vi "Main.vi"() -> ()   [LabVIEW 2017]
uses:
  47dd9ab8-544f-4192-a7de-fb61588ea7e2.vi
panel:
  out "Thermometer m6":dbl(slide) scale=10.0..50.0
  out "Thermometer m5":dbl(slide) scale=10.0..50.0
  out "Thermometer m3":dbl(slide) scale=10.0..50.0
  out "Thermometer m2":dbl(slide) scale=10.0..50.0
  out "Load m6":dbl(knob) scale=0.0..50.0
  out "Load m5":dbl(knob) scale=0.0..50.0
  out "Load m3":dbl(knob) scale=0.0..50.0
  out "Load m2":dbl(knob) scale=0.0..50.0
  out "error out":errorcluster
  in  "error in (no error)":errorcluster
  in  "Color m6":T1(ring)
  in  "Color m5":T1(ring)
  in  "Color m3":T1(ring)
  in  "Color m2":T1(ring)
  in  "Speed m6":dbl(slide)=1.0 scale=0.2..2.0
  in  "Speed m5":dbl(slide)=1.0 scale=0.2..2.0
  in  "Speed m3":dbl(slide)=1.0 scale=0.2..2.0
  in  "Speed m2":dbl(slide)=1.0 scale=0.2..2.0
  in  "m6":dbl(knob) scale=-23.0..90.0
  in  "m5":dbl(knob) scale=-90.0..90.0
  in  "m3":dbl(knob) scale=-90.0..90.0
  in  "m2":dbl(knob) scale=-90.0..90.0
  in  "stop":bool
  out "Picture":picture
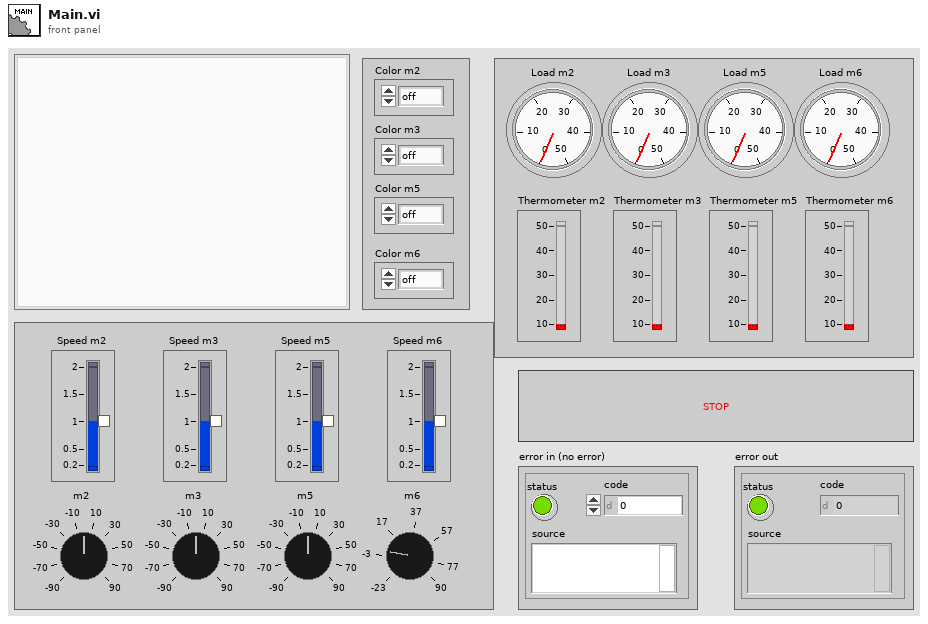
[diagram p1: front panel]
types:
  T1 = enum16{"off", "red", "green", "yellow", "blue", "pink", "cyan", "white"}
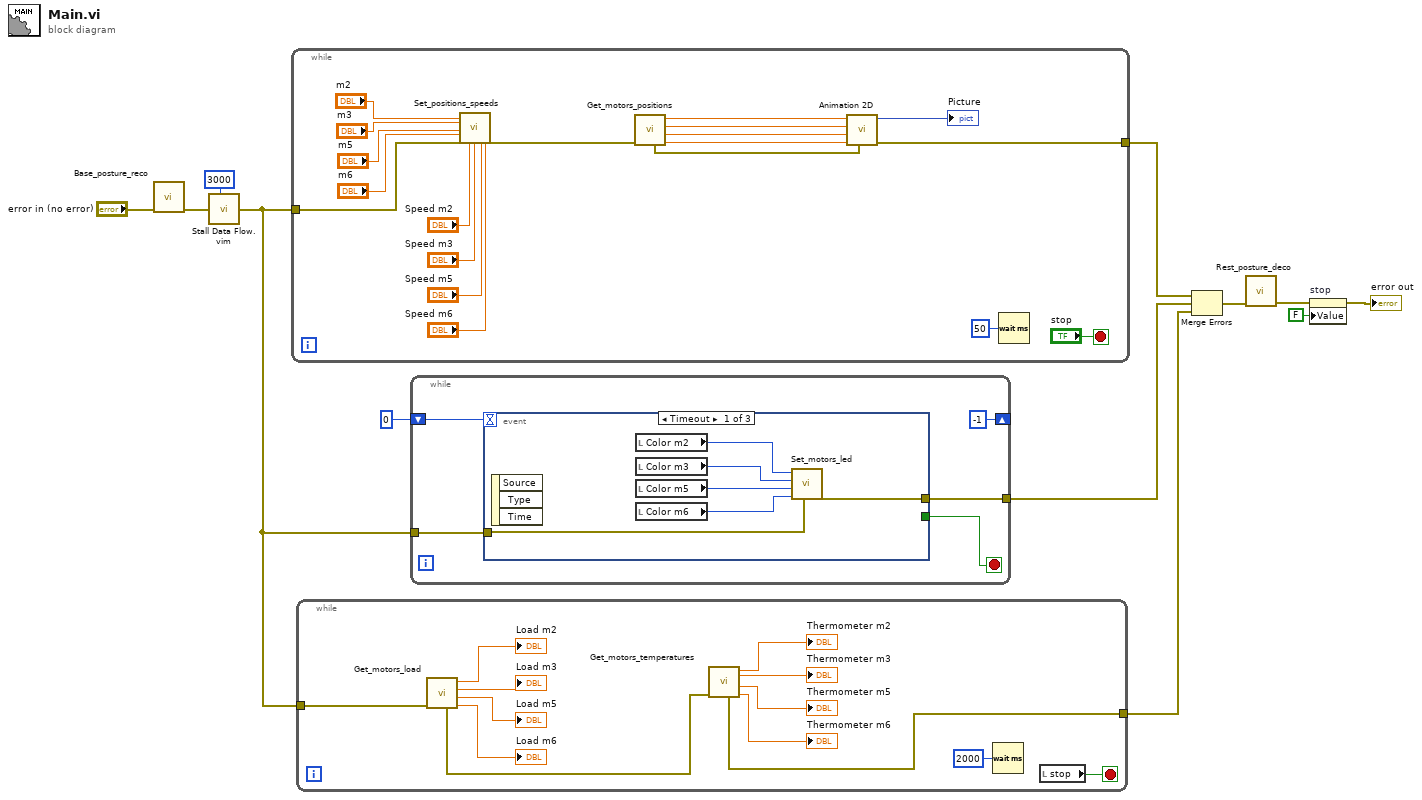
[diagram p0: block diagram]
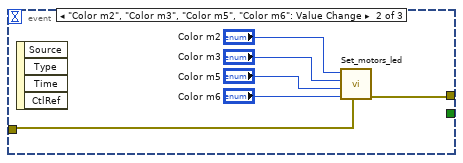
[diagram p2: hidden frame]
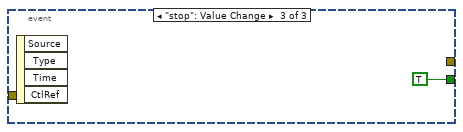
[diagram p3: hidden frame]
diagram:
  n1 = call "Base_posture_reco.vi"("error in (no error)"="error in (no error)") -> ("error out"=w5:errorcluster)  [unwired: 10 in]
  n2 = call "Stall Data Flow.vim"("value in"=w5, "milliseconds to wait"=u32 3000) -> ("value out"=w3:errorcluster)  [unwired: 1 out]
  n3 = while {
    tunnel: w3 -> [w16]
    tunnel: [w13] -> w11
    stop <- "stop" stop-if-true
    n4 = call "Set_positions_speeds.vi"("m2"="m2", "m3"="m3", "m5"="m5", "m6"="m6", "error in (no error)"=w16, "Speed m2"="Speed m2", "Speed m3"="Speed m3", "Speed m5"="Speed m5", "Speed m6"="Speed m6") -> ("error out"=w15:errorcluster)  [unwired: 18 in]
    n5 = call "Get_motors_positions.vi"("error in (no error)"=w15) -> ("m6"=w28:dbl, "m5"=w29:dbl, "m3"=w30:dbl, "m2"=w31:dbl, "error out"=w14:errorcluster)  [unwired: 6 in]
    n6 = call "Animation 2D.vi"("m2"=w31, "m3"=w30, "m5"=w29, "m6"=w28, "error in (no error)"=w14) -> ("Picture"=→"Picture":picture, "error out"=w13:errorcluster)  [unwired: 4 in]
    n7 = Wait (ms)(milliseconds to wait=u32 50) -> ()  [unwired: 1 out]
  }
  n8 = while {
    tunnel: w3 -> [w40]
    tunnel: [w36] -> w9
    stop <- w39 stop-if-true
    n9 = call "Get_motors_load.vi"("error in (no error)"=w40) -> ("m6"=→"Load m6":dbl, "m5"=→"Load m5":dbl, "m3"=→"Load m3":dbl, "m2"=→"Load m2":dbl, "error out"=w37:errorcluster)  [unwired: 6 in]
    n10 = call "Get_motors_temperatures.vi"("error in (no error)"=w37) -> ("m6"=→"Thermometer m6":dbl, "m5"=→"Thermometer m5":dbl, "m3"=→"Thermometer m3":dbl, "m2"=→"Thermometer m2":dbl, "error out"=w36:errorcluster)  [unwired: 6 in]
    n11 = Wait (ms)(milliseconds to wait=u32 2000) -> ()  [unwired: 1 out]
    n12 = local read "stop"() -> (w39:bool)
  }
  n13 = while {
    shift-right: [-1] -> _
    shift-left: 0 -> [w49]
    tunnel: [w47] -> w10
    tunnel: w3 -> [w46]
    stop <- w45 stop-if-true
    n14 = event shown="[0] Timeout" {
      selector: _ -> [_ _ _]
      dyn-events: _ -> [_ _ _]
      timeout: w49 -> [_ _ _]
      tunnel: [w51 w57 _] -> w47
      tunnel: w46 -> [w50 w58 _]
      tunnel: [_ _ TRUE] -> w45
      event Timeout {
        n15 = event-data() -> ()  [unwired: 1 in, 3 out]
        n16 = local read "Color m2"() -> (w55:T1)
        n17 = local read "Color m3"() -> (w54:T1)
        n18 = local read "Color m5"() -> (w53:T1)
        n19 = local read "Color m6"() -> (w52:T1)
        n20 = call "Set_motors_led.vi"("error in (no error)"=w50, "Color m6"=w52, "Color m5"=w53, "Color m3"=w54, "Color m2"=w55) -> ("error out"=w51:errorcluster)  [unwired: 6 in]
      }
      event "Color m2", "Color m3", "Color m5", "Color m6": Value Change {
        n21 = event-data() -> ()  [unwired: 1 in, 4 out]
        n22 = call "Set_motors_led.vi"("error in (no error)"=w58, "Color m6"="Color m6", "Color m5"="Color m5", "Color m3"="Color m3", "Color m2"="Color m2") -> ("error out"=w57:errorcluster)  [unwired: 6 in]
      }
      event "stop": Value Change {
        n23 = event-data() -> ()  [unwired: 1 in, 4 out]
      }
    }
  }
  n24 = Merge Errors(w11, w10, w9) -> (w2:errorcluster)
  n25 = call "Rest_posture_deco.vi"("error in (no error)"=w2) -> ("error out"=w1:errorcluster)  [unwired: 10 in]
  n26 = property on="stop" class="Bool (strict)"(error in=w1, "Value"=FALSE ("stop")) -> (error out=→"error out":errorcluster)  [unwired: 1 in, 1 out]
